vi "Cycle_Calculator.vi"(7 "Cycle Specs":T1, 8 "Excitation Specs":T2) -> (0 "Samples Before Frequency Change":i32[](array[numeric]), 1 "Samples Before Measuring":i32[](array[numeric]), 2 "Samples Needed to Settle":i32[](array[numeric]), 3 "Samples for Calculation":i32[](array[numeric]), 5 "Excitation Frequencies":dbl[](array[numeric]), 6 "Total Number of Samples":i32)   [LabVIEW 2020, in "DynamicSignalAnalyzer.lvlib"]
doc: "Calculates a list of logmartically spaced frequencies to excite the system at, the number of samples needed to be ignored in waiting for the excitation to settle and the number of samples needed to be measured in order to calculate the frequency response for each excitation frequency.\n\nInputs: \n\n- Excitation Specs:\n - Used: Initial Frequency, Final Frequency, Frequency Units, Number of Frequencies, & Sampling Time\n - Not: Amplitude & Offset\n\n- Cycle Specs\n - Used: Cycles to Settle & Cycles to Calculate\n\nOutputs:\n\n- Excitation Frequencies: A list of logmarithically spaced frequencies to excite the system at.\n\n- Samples for Calculation: A list of the number of samples to be measured per frequency to measure the freqeuncy response.\n\n- Samples Needed to Settle: A list of the number of samples to ignore in waiting for the system to settle\n\n- Samples Before Freq. Change: A list of the indices of the last sample taken at a particular frequency before the frequency changes. The following sample, the excitaton frequency changes. \n\n- Samples Before Measuring: A list of the last sample ingored. The following sample, measuring should begin.\n\n- Total Number of Samples: The total samples (ingored + measured) needed to run the DSA."
uses:
  DynamicSignalAnalyzer.lvlib
  <vilib>/Analysis/1siggen.llb/Ramp Pattern by Samples.vi
  <vilib>/Analysis/NI_AALBase.lvlib
panel:
  # "Cycle_Calculator"
  # "DSA Specs"
  # "Outputs"
  # "Excitation Frequencies"
  # "Samples Needed"
  # "Measuring"
  # "Frequency Change"
  # "Per Frequency"
  # "Per Frequency"
  # "Excitation Frequencies"
  # "Frequency\nUnits"
  # "[Hz]"
  # "Excitation Magnitude"
  # "[rad/s]"
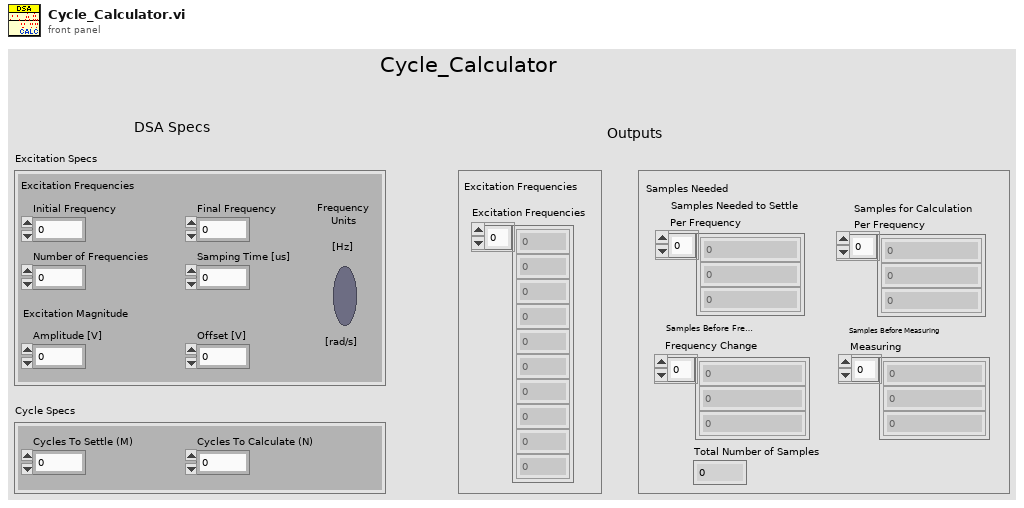
[diagram p1: front panel]
types:
  T1 = cluster{"Cycles To Settle (M)":i16, "Cycles To Calculate (N)":i16}
  T2 = cluster{"Initial Frequency":dbl, "Final Frequency":dbl, "Number of Frequencies":i16, "Samping Time [us]":dbl, "Amplitude [V]":dbl, "Offset [V]":dbl, "Freq Unit":bool}
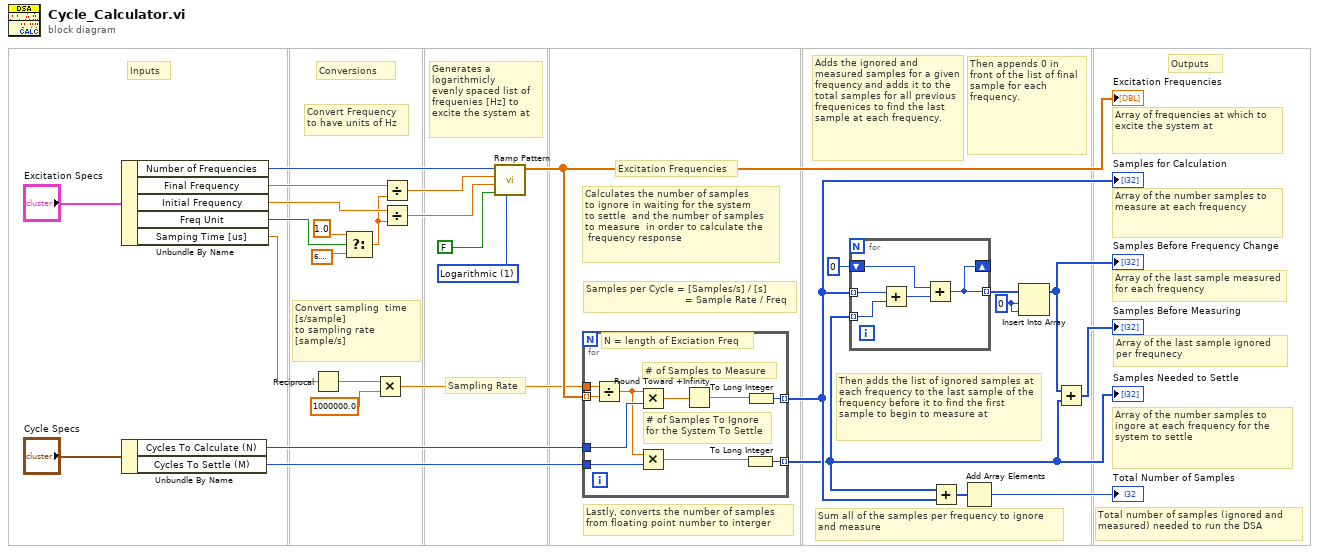
[diagram p0: block diagram]
diagram:
  w7 = 0
  w18 = u16 1 items=["Linear", "Logarithmic"] ("type")
  # "Then appends 0 in front of the list of final sample for each frequency."
  # "Then adds the list of ignored samples at each frequency to the last sample of the frequency before it to find the first sample to begin to measure at"
  # "Array of the last sample ignored per frequnecy"
  # "Adds the ignored and measured samples for a given frequency and adds it to the total samples for all previous frequenices to find the last sample at each frequency."
  # "Sum all of the samples per frequency to ignore and measure"
  # "Total number of samples (ignored and measured) needed to run the DSA"
  # "Array of the last sample measured for each frequency"
  # "Array of the number samples to ingore at each frequency for the system to settle"
  # "Array of the number samples to measure at each frequency"
  # "Array of frequencies at which to excite the system at"
  # "Lastly, converts the number of samples\nfrom floating point number to interger"
  # "Sampling Rate"
  # "Samples per Cycle = [Samples/s] / [s]\n                                 = Sample Rate / Freq"
  # "Excitation Frequencies"
  # "Outputs"
  # "Calculates the number of samples \nto ignore in waiting for the system \nto settle  and the number of samples\nto measure  in order to calculate the\n frequency response"
  # "Convert sampling  time\n[s/sample]\nto sampling rate \n[sample/s]"
  # "Conversions"
  # "Generates a\nlogarithmicly\nevenly spaced list of \nfrequenies [Hz] to\nexcite the system at"
  # "Inputs"
  # "Convert Frequency\nto have units of Hz"
  n1 = Unbundle By Name("Excitation Specs") -> ("Number of Frequencies"=w28:i16, "Final Frequency"=w27:dbl, "Initial Frequency"=w26:dbl, "Freq Unit"=w23:bool, "Samping Time [us]"=w16:dbl)
  n2 = Unbundle By Name("Cycle Specs") -> ("Cycles To Calculate (N)"=w15:i16, "Cycles To Settle (M)"=w14:i16)
  n3 = Reciprocal(x=w16) -> (1/x=w3:dbl)
  n4 = Select(t=1.0, s=w23, f=6.283185307179586) -> (s? t:f=w22:dbl)
  n5 = Multiply(x=w3, y=1000000.0) -> (x*y=w2:dbl)
  n6 = Divide(x=w27, y=w22) -> (x/y=w21:dbl)
  n7 = Divide(x=w26, y=w22) -> (x/y=w20:dbl)
  n8 = call-poly <vilib>:"Ramp Pattern.vi"("type"=w18, "exclude end?"=FALSE, "start"=w20, "end"=w21, "samples"=w28) -> ("Ramp Pattern"=w9:dbl[])  [unwired: 5 in, 1 out]
  "Excitation Frequencies" <- w9
  n9 = for {
    tunnel: w9 -> [w39] mode=indexing
    tunnel: w2 -> [w38]
    tunnel: w15 -> [w37]
    tunnel: w14 -> [w35]
    tunnel: [w31] -> w10 mode=indexing
    tunnel: [w30] -> w6 mode=indexing
    # "# of Samples To Ignore\nfor the System To Settle"
    # "# of Samples to Measure"
    # "N = length of Exciation Freq"
    n10 = Divide(x=w38, y=w39) -> (x/y=w36:dbl)
    n11 = Multiply(x=w36, y=w37) -> (x*y=w34:dbl)
    n12 = Multiply(x=w36, y=w35) -> (x*y=w32:dbl)
    n13 = Round Toward +Infinity(x=w34) -> (ceil(x): smallest int >= x=w33:dbl)
    n14 = To Long Integer(number=w32) -> (32bit integer=w30:i32)
    n15 = To Long Integer(number=w33) -> (32bit integer=w31:i32)
  }
  "Samples for Calculation" <- w10
  "Samples Needed to Settle" <- w6
  n16 = for {
    shift-right: [w40] -> _
    shift-left: 0 -> [w41]
    tunnel: w10 -> [w44] mode=indexing
    tunnel: w6 -> [w43] mode=indexing
    tunnel: [w40] -> w8 mode=indexing
    n17 = Add(x=w44, y=w43) -> (x+y=w42:i32)
    n18 = Add(x=w41, y=w42) -> (x+y=w40:i32)
  }
  n19 = Add(x=w6, y=w10) -> (x+y=w13:i32[])
  n20 = Add Array Elements(numeric array=w13) -> (sum=→"Total Number of Samples":i32)
  n21 = Insert Into Array(array=w8, index=w7, new element=w7) -> (w5:i32[])
  "Samples Before Frequency Change" <- w5
  n22 = Add(x=w5, y=w6) -> (x+y=→"Samples Before Measuring":i32[])
